vi "DB_修改通讯表.vi"(8 "error in (no error)":errorcluster caption="错误输入（无错误）", 9 "设备通讯参数":T1={"Unit ID"=1, "IP Address"="127.0.0.1", "Port"=255, "Serial Port"="COM3", "baud rate (9600)"=9600, "Protocol"=enum."Serial Port"}, 10 "id":i32, 11 "SQLite Connection in":refnum<class "Connection.lvclass">) -> (0 "error out":errorcluster caption="错误输出", 3 "SQLite Connection":refnum<class "Connection.lvclass">)   [LabVIEW 2018]
uses:
  <vilib>/drjdpowell/SQLite Library/SQL Connection/Connection.lvclass
  <vilib>/drjdpowell/SQLite Library/SQL Statement/SQL Statement.lvclass/SQL Statement.ctl
  <vilib>/drjdpowell/SQLite Library/SQL Connection/Open (path).vi
  <vilib>/drjdpowell/SQLite Library/SQL Statement/Bind Text.vi
  <vilib>/drjdpowell/SQLite Library/SQL Statement/Bind Integer.vi
  <vilib>/drjdpowell/SQLite Library/SQL Connection/Open (string).vi
  <vilib>/drjdpowell/SQLite Library/SQL Statement/Step.vi
  <vilib>/AdvancedString/Path To Command Line String.vi
  <vilib>/drjdpowell/SQLite Library/SQL Statement/Error Message.vi
  <vilib>/drjdpowell/SQLite Library/SQL Statement/SQL Statement.lvclass
  <vilib>/drjdpowell/SQLite Library/Transaction Helpers/Transaction.lvlib
panel:
  out "连接的字符串":string
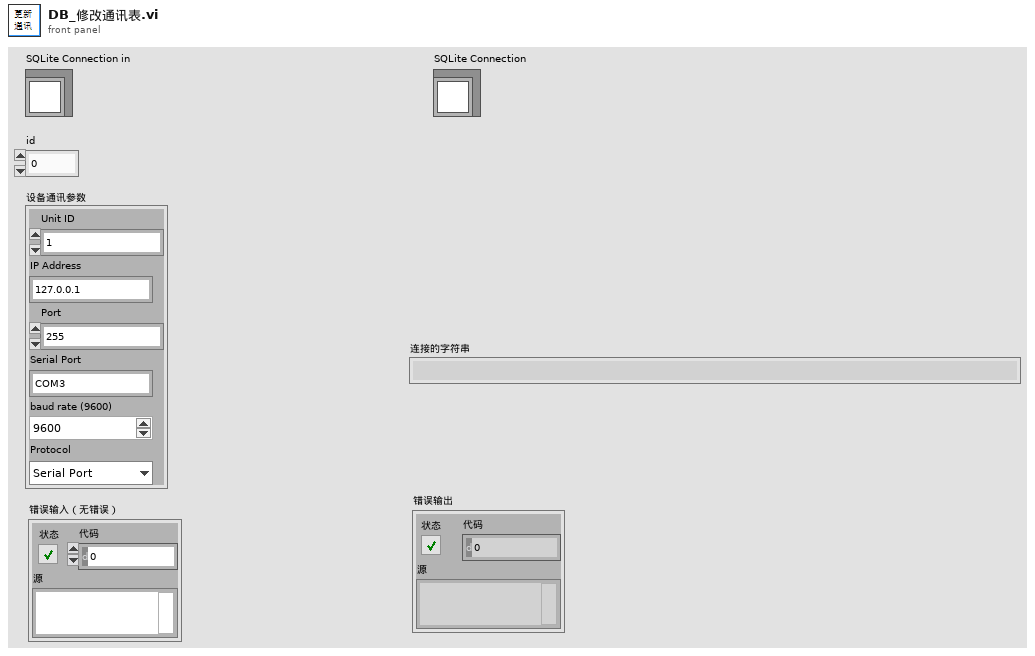
[diagram p1: front panel]
types:
  T1 = cluster{"Unit ID":u8, "IP Address":string, "Port":u16, "Serial Port":string, "baud rate (9600)":u32, "Protocol":enum16{"Serial Port", "Modbus TCP/IP"}}
  T2 = enum16{"New or existing", "Existing", "Read only"}
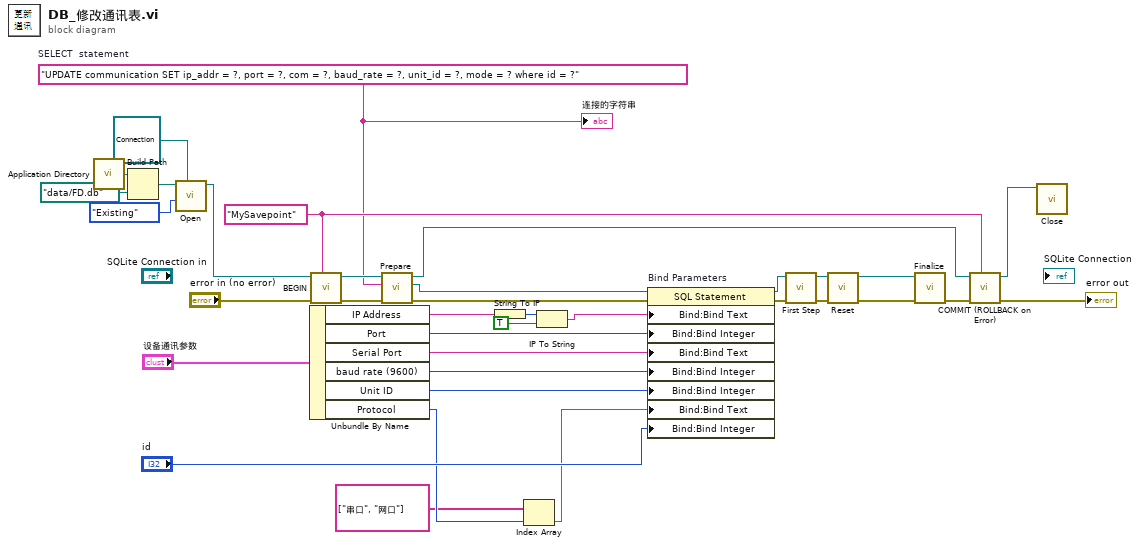
[diagram p0: block diagram]
diagram:
  w34 = "MySavepoint" ("Savepoint name")
  w27 = "UPDATE communication SET ip_addr = ?, port = ?, com = ?, baud_rate = ?, unit_id = ?, mode = ? where id = ?"  # SELECT  statement
  n1 = call <vilib>:"Application Directory.vi"() -> ("Application Directory"=w11:path)
  n2 = Build Path(base path=w11, name or relative path=path "data/FD.db" ("Application Directory")) -> (appended path=w9:path)
  n3 = call-poly <vilib>:"Open.vi"("SQLite Connection type"=refnum<class "Connection.lvclass"> refnum, "File Option"=T2."Existing", "db file"=w9) -> ("SQLite Connection"=w6:refnum<class "Connection.lvclass">)  [unwired: 7 in, 1 out]
  n4 = Unbundle By Name("设备通讯参数") -> ("IP Address"=w1:string, "Port"=w20:u16, "Serial Port"=w19:string, "baud rate (9600)"=w17:u32, "Unit ID"=w16:u8, "Protocol"=w14:enum16{"Serial Port", "Modbus TCP/IP"})
  n5 = call <vilib>:"BEGIN.vi"("Savepoint name"=w34, "error in (no error)"="error in (no error)", "SQLite Connection in"=w6) -> ("error out"=w33:errorcluster, "SQLite Connection"=w32:refnum<class "Connection.lvclass">)  [unwired: 7 in]
  n6 = call <vilib>:"Prepare.vi"("error in (no error)"=w33, "SQL"=w27, "SQLite Connection in"=w32) -> ("error out"=w29:errorcluster, "SQL Statement"=w28:refnum<class "SQL Statement.lvclass">, "SQLite Connection"=w35:refnum<class "Connection.lvclass">)  [unwired: 4 in, 2 out]
  n7 = String To IP(1:w1) -> (0:w3:u32)
  n8 = Index Array(array=string[] ["串口", "网口"], index=w14) -> (element=w13:string)
  n9 = IP To String(1:TRUE ("句点符号？(F)"), 2:w3) -> (0:w2:string)
  n10 = property on="Bind Parameters" class="SQL Statement"(reference=w28, error in=w29, "Bind:Bind Text"=w2, "Bind:Bind Integer"=w20, "Bind:Bind Text"=w19, "Bind:Bind Integer"=w17, "Bind:Bind Integer"=w16, "Bind:Bind Text"=w13, "Bind:Bind Integer"="id") -> (reference out=w26:refnum<class "SQL Statement.lvclass">, error out=w25:errorcluster)
  n11 = call <vilib>:"First Step.vi"("error in (no error)"=w25, "SQL Statement in"=w26) -> ("error out"=w24:errorcluster, "SQL Statement"=w23:refnum<class "SQL Statement.lvclass">)  [unwired: 7 in, 1 out]
  n12 = call <vilib>:"Reset.vi"("error in (no error)"=w24, "SQL Statement in"=w23) -> ("error out"=w31:errorcluster, "SQL Statement"=w30:refnum<class "SQL Statement.lvclass">)  [unwired: 8 in]
  n13 = call <vilib>:"Finalize.vi"("error in (no error)"=w31, "SQL Statement in"=w30) -> ("error out"=w36:errorcluster)  [unwired: 9 in]
  n14 = call <vilib>:"COMMIT (ROLLBACK on Error).vi"("Savepoint name"=w34, "error in (no error)"=w36, "SQLite Connection in"=w35) -> ("error out"=→"error out":errorcluster, "SQLite Connection"=w5:refnum<class "Connection.lvclass">)  [unwired: 7 in]
  n15 = call-dynamic "Close.vi"("SQLite Connection in"=w5) -> ()  [unwired: 10 in, 1 out]
  "连接的字符串" <- w27
